vi "FipsAdjacent.vi"() -> (11 "Fips":i32[](array[numeric]))   [LabVIEW 2017] (continued)
CA\"\t06005\t\"El Dorado County, CA\"\t06017\n\"Amador County, CA\"\t06005\t\"Sacramento County, CA\"\t06067\n\"Amador County, CA\"\t06005\t\"San Joaquin County, CA\"\t06077\n\"Butte County, CA\"\t06007\t\"Butte County, CA\"\t06007\n\"Butte County, CA\"\t06007\t\"Colusa County, CA\"\t06011\n\"Butte County, CA\"\t06007\t\"Glenn County, CA\"\t06021\n\"Butte County, CA\"\t06007\t\"Plumas County, CA\"\t06063\n\"Butte County, CA\"\t06007\t\"Sutter County, CA\"\t06101\n\"Butte County, CA\"\t06007\t\"Tehama County, CA\"\t06103\n\"Butte County, CA\"\t06007\t\"Yuba County, CA\"\t06115\n\"Calaveras County, CA\"\t06009\t\"Alpine County, CA\"\t06003\n\"Calaveras County, CA\"\t06009\t\"Amador County, CA\"\t06005\n\"Calaveras County, CA\"\t06009\t\"Calaveras County, CA\"\t06009\n\"Calaveras County, CA\"\t06009\t\"San Joaquin County, CA\"\t06077\n\"Calaveras County, CA\"\t06009\t\"Stanislaus County, CA\"\t06099\n\"Calaveras County, CA\"\t06009\t\"Tuolumne County, CA\"\t06109\n\"Colusa County, CA\"\t06011\t\"Butte County, CA\"\t06007\n\"Colusa County, CA\"\t06011\t\"Colusa County, CA\"\t06011\n\"Colusa County, CA\"\t06011\t\"Glenn County, CA\"\t06021\n\"Colusa County, CA\"\t06011\t\"Lake County, CA\"\t06033\n\"Colusa County, CA\"\t06011\t\"Sutter County, CA\"\t06101\n\"Colusa County, CA\"\t06011\t\"Yolo County, CA\"\t06113\n\"Contra Costa County, CA\"\t06013\t\"Alameda County, CA\"\t06001\n\"Contra Costa County, CA\"\t06013\t\"Contra Costa County, CA\"\t06013\n\"Contra Costa County, CA\"\t06013\t\"Marin County, CA\"\t06041\n\"Contra Costa County, CA\"\t06013\t\"Sacramento County, CA\"\t06067\n\"Contra Costa County, CA\"\t06013\t\"San Francisco County, CA\"\t06075\n\"Contra Costa County, CA\"\t06013\t\"San Joaquin County, CA\"\t06077\n\"Contra Costa County, CA\"\t06013\t\"Solano County, CA\"\t06095\n\"Contra Costa County, CA\"\t06013\t\"Sonoma County, CA\"\t06097\n\"Del Norte County, CA\"\t06015\t\"Del Norte County, CA\"\t06015\n\"Del Norte County, CA\"\t06015\t\"Humboldt County, CA\"\t06023\n\"Del Norte County, CA\"\t06015\t\"Siskiyou County, CA\"\t06093\n\"Del Norte County, CA\"\t06015\t\"Curry County, OR\"\t41015\n\"Del Norte County, CA\"\t06015\t\"Josephine County, OR\"\t41033\n\"El Dorado County, CA\"\t06017\t\"Alpine County, CA\"\t06003\n\"El Dorado County, CA\"\t06017\t\"Amador County, CA\"\t06005\n\"El Dorado County, CA\"\t06017\t\"El Dorado County, CA\"\t06017\n\"El Dorado County, CA\"\t06017\t\"Placer County, CA\"\t06061\n\"El Dorado County, CA\"\t06017\t\"Sacramento County, CA\"\t06067\n\"El Dorado County, CA\"\t06017\t\"Douglas County, NV\"\t32005\n\"Fresno County, CA\"\t06019\t\"Fresno County, CA\"\t06019\n\"Fresno County, CA\"\t06019\t\"Inyo County, CA\"\t06027\n\"Fresno County, CA\"\t06019\t\"Kings County, CA\"\t06031\n\"Fresno County, CA\"\t06019\t\"Madera County, CA\"\t06039\n\"Fresno County, CA\"\t06019\t\"Merced County, CA\"\t06047\n\"Fresno County, CA\"\t06019\t\"Mono County, CA\"\t06051\n\"Fresno County, CA\"\t06019\t\"Monterey County, CA\"\t06053\n\"Fresno County, CA\"\t06019\t\"San Benito County, CA\"\t06069\n\"Fresno County, CA\"\t06019\t\"Tulare County, CA\"\t06107\n\"Glenn County, CA\"\t06021\t\"Butte County, CA\"\t06007\n\"Glenn County, CA\"\t06021\t\"Colusa County, CA\"\t06011\n\"Glenn County, CA\"\t06021\t\"Glenn County, CA\"\t06021\n\"Glenn County, CA\"\t06021\t\"Lake County, CA\"\t06033\n\"Glenn County, CA\"\t06021\t\"Mendocino County, CA\"\t06045\n\"Glenn County, CA\"\t06021\t\"Tehama County, CA\"\t06103\n\"Humboldt County, CA\"\t06023\t\"Del Norte County, CA\"\t06015\n\"Humboldt County, CA\"\t06023\t\"Humboldt County, CA\"\t06023\n\"Humboldt County, CA\"\t06023\t\"Mendocino County, CA\"\t06045\n\"Humboldt County, CA\"\t06023\t\"Siskiyou County, CA\"\t06093\n\"Humboldt County, CA\"\t06023\t\"Trinity County, CA\"\t06105\n\"Imperial County, CA\"\t06025\t\"La Paz County, AZ\"\t04012\n\"Imperial County, CA\"\t06025\t\"Yuma County, AZ\"\t04027\n\"Imperial County, CA\"\t06025\t\"Imperial County, CA\"\t06025\n\"Imperial County, CA\"\t06025\t\"Riverside County, CA\"\t06065\n\"Imperial County, CA\"\t06025\t\"San Diego County, CA\"\t06073\n\"Inyo County, CA\"\t06027\t\"Fresno County, CA\"\t06019\n\"Inyo County, CA\"\t06027\t\"Inyo County, CA\"\t06027\n\"Inyo County, CA\"\t06027\t\"Kern County, CA\"\t06029\n\"Inyo County, CA\"\t06027\t\"Mono County, CA\"\t06051\n\"Inyo County, CA\"\t06027\t\"San Bernardino County, CA\"\t06071\n\"Inyo County, CA\"\t06027\t\"Tulare County, CA\"\t06107\n\"Inyo County, CA\"\t06027\t\"Clark County, NV\"\t32003\n\"Inyo County, CA\"\t06027\t\"Esmeralda County, NV\"\t32009\n\"Inyo County, CA\"\t06027\t\"Nye County, NV\"\t32023\n\"Kern County, CA\"\t06029\t\"Inyo County, CA\"\t06027\n\"Kern County, CA\"\t06029\t\"Kern County, CA\"\t06029\n\"Kern County, CA\"\t06029\t\"Kings County, CA\"\t06031\n\"Kern County, CA\"\t06029\t\"Los Angeles County, CA\"\t06037\n\"Kern County, CA\"\t06029\t\"San Bernardino County, CA\"\t06071\n\"Kern County, CA\"\t06029\t\"San Luis Obispo County, CA\"\t06079\n\"Kern County, CA\"\t06029\t\"Santa Barbara County, CA\"\t06083\n\"Kern County, CA\"\t06029\t\"Tulare County, CA\"\t06107\n\"Kern County, CA\"\t06029\t\"Ventura County, CA\"\t06111\n\"Kings County, CA\"\t06031\t\"Fresno County, CA\"\t06019\n\"Kings County, CA\"\t06031\t\"Kern County, CA\"\t06029\n\"Kings County, CA\"\t06031\t\"Kings County, CA\"\t06031\n\"Kings County, CA\"\t06031\t\"Monterey County, CA\"\t06053\n\"Kings County, CA\"\t06031\t\"San Luis Obispo County, CA\"\t06079\n\"Kings County, CA\"\t06031\t\"Tulare County, CA\"\t06107\n\"Lake County, CA\"\t06033\t\"Colusa County, CA\"\t06011\n\"Lake County, CA\"\t06033\t\"Glenn County, CA\"\t06021\n\"Lake County, CA\"\t06033\t\"Lake County, CA\"\t06033\n\"Lake County, CA\"\t06033\t\"Mendocino County, CA\"\t06045\n\"Lake County, CA\"\t06033\t\"Napa County, CA\"\t06055\n\"Lake County, CA\"\t06033\t\"Sonoma County, CA\"\t06097\n\"Lake County, CA\"\t06033\t\"Yolo County, CA\"\t06113\n\"Lassen County, CA\"\t06035\t\"Lassen County, CA\"\t06035\n\"Lassen County, CA\"\t06035\t\"Modoc County, CA\"\t06049\n\"Lassen County, CA\"\t06035\t\"Plumas County, CA\"\t06063\n\"Lassen County, CA\"\t06035\t\"Shasta County, CA\"\t06089\n\"Lassen County, CA\"\t06035\t\"Sierra County, CA\"\t06091\n\"Lassen County, CA\"\t06035\t\"Washoe County, NV\"\t32031\n\"Los Angeles County, CA\"\t06037\t\"Kern County, CA\"\t06029\n\"Los Angeles County, CA\"\t06037\t\"Los Angeles County, CA\"\t06037\n\"Los Angeles County, CA\"\t06037\t\"Orange County, CA\"\t06059\n\"Los Angeles County, CA\"\t06037\t\"San Bernardino County, CA\"\t06071\n\"Los Angeles County, CA\"\t06037\t\"Ventura County, CA\"\t06111\n\"Madera County, CA\"\t06039\t\"Fresno County, CA\"\t06019\n\"Madera County, CA\"\t06039\t\"Madera County, CA\"\t06039\n\"Madera County, CA\"\t06039\t\"Mariposa County, CA\"\t06043\n\"Madera County, CA\"\t06039\t\"Merced County, CA\"\t06047\n\"Madera County, CA\"\t06039\t\"Mono County, CA\"\t06051\n\"Madera County, CA\"\t06039\t\"Tuolumne County, CA\"\t06109\n\"Marin County, CA\"\t06041\t\"Contra Costa County, CA\"\t06013\n\"Marin County, CA\"\t06041\t\"Marin County, CA\"\t06041\n\"Marin County, CA\"\t06041\t\"San Francisco County, CA\"\t06075\n\"Marin County, CA\"\t06041\t\"Solano County, CA\"\t06095\n\"Marin County, CA\"\t06041\t\"Sonoma County, CA\"\t06097\n\"Mariposa County, CA\"\t06043\t\"Madera County, CA\"\t06039\n\"Mariposa County, CA\"\t06043\t\"Mariposa County, CA\"\t06043\n\"Mariposa County, CA\"\t06043\t\"Merced County, CA\"\t06047\n\"Mariposa County, CA\"\t06043\t\"Stanislaus County, CA\"\t06099\n\"Mariposa County, CA\"\t06043\t\"Tuolumne County, CA\"\t06109\n\"Mendocino County, CA\"\t06045\t\"Glenn County, CA\"\t06021\n\"Mendocino County, CA\"\t06045\t\"Humboldt County, CA\"\t06023\n\"Mendocino County, CA\"\t06045\t\"Lake County, CA\"\t06033\n\"Mendocino County, CA\"\t06045\t\"Mendocino County, CA\"\t06045\n\"Mendocino County, CA\"\t06045\t\"Sonoma County, CA\"\t06097\n\"Mendocino County, CA\"\t06045\t\"Tehama County, CA\"\t06103\n\"Mendocino County, CA\"\t06045\t\"Trinity County, CA\"\t06105\n\"Merced County, CA\"\t06047\t\"Fresno County, CA\"\t06019\n\"Merced County, CA\"\t06047\t\"Madera County, CA\"\t06039\n\"Merced County, CA\"\t06047\t\"Mariposa County, CA\"\t06043\n\"Merced County, CA\"\t06047\t\"Merced County, CA\"\t06047\n\"Merced County, CA\"\t06047\t\"San Benito County, CA\"\t06069\n\"Merced County, CA\"\t06047\t\"Santa Clara County, CA\"\t06085\n\"Merced County, CA\"\t06047\t\"Stanislaus County, CA\"\t06099\n\"Modoc County, CA\"\t06049\t\"Lassen County, CA\"\t06035\n\"Modoc County, CA\"\t06049\t\"Modoc County, CA\"\t06049\n\"Modoc County, CA\"\t06049\t\"Shasta County, CA\"\t06089\n\"Modoc County, CA\"\t06049\t\"Siskiyou County, CA\"\t06093\n\"Modoc County, CA\"\t06049\t\"Washoe County, NV\"\t32031\n\"Modoc County, CA\"\t06049\t\"Klamath County, OR\"\t41035\n\"Modoc County, CA\"\t06049\t\"Lake County, OR\"\t41037\n\"Mono County, CA\"\t06051\t\"Alpine County, CA\"\t06003\n\"Mono County, CA\"\t06051\t\"Fresno County, CA\"\t06019\n\"Mono County, CA\"\t06051\t\"Inyo County, CA\"\t06027\n\"Mono County, CA\"\t06051\t\"Madera County, CA\"\t06039\n\"Mono County, CA\"\t06051\t\"Mono County, CA\"\t06051\n\"Mono County, CA\"\t06051\t\"Tuolumne County, CA\"\t06109\n\"Mono County, CA\"\t06051\t\"Douglas County, NV\"\t32005\n\"Mono County, CA\"\t06051\t\"Esmeralda County, NV\"\t32009\n\"Mono County, CA\"\t06051\t\"Lyon County, NV\"\t32019\n\"Mono County, CA\"\t06051\t\"Mineral County, NV\"\t32021\n\"Monterey County, CA\"\t06053\t\"Fresno County, CA\"\t06019\n\"Monterey County, CA\"\t06053\t\"Kings County, CA\"\t06031\n\"Monterey County, CA\"\t06053\t\"Monterey County, CA\"\t06053\n\"Monterey County, CA\"\t06053\t\"San Benito County, CA\"\t06069\n\"Monterey County, CA\"\t06053\t\"San Luis Obispo County, CA\"\t06079\n\"Monterey County, CA\"\t06053\t\"Santa Cruz County, CA\"\t06087\n\"Napa County, CA\"\t06055\t\"Lake County, CA\"\t06033\n\"Napa County, CA\"\t06055\t\"Napa County, CA\"\t06055\n\"Napa County, CA\"\t06055\t\"Solano County, CA\"\t06095\n\"Napa County, CA\"\t06055\t\"Sonoma County, CA\"\t06097\n\"Napa County, CA\"\t06055\t\"Yolo County, CA\"\t06113\n\"Nevada County, CA\"\t06057\t\"Nevada County, CA\"\t06057\n\"Nevada County, CA\"\t06057\t\"Placer County, CA\"\t06061\n\"Nevada County, CA\"\t06057\t\"Sierra County, CA\"\t06091\n\"Nevada County, CA\"\t06057\t\"Yuba County, CA\"\t06115\n\"Nevada County, CA\"\t06057\t\"Washoe County, NV\"\t32031\n\"Orange County, CA\"\t06059\t\"Los Angeles County, CA\"\t06037\n\"Orange County, CA\"\t06059\t\"Orange County, CA\"\t06059\n\"Orange County, CA\"\t06059\t\"Riverside County, CA\"\t06065\n\"Orange County, CA\"\t06059\t\"San Bernardino County, CA\"\t06071\n\"Orange County, CA\"\t06059\t\"San Diego County, CA\"\t06073\n\"Placer County, CA\"\t06061\t\"El Dorado County, CA\"\t06017\n\"Placer County, CA\"\t06061\t\"Nevada County, CA\"\t06057\n\"Placer County, CA\"\t06061\t\"Placer County, CA\"\t06061\n\"Placer County, CA\"\t06061\t\"Sacramento County, CA\"\t06067\n\"Placer County, CA\"\t06061\t\"Sutter County, CA\"\t06101\n\"Placer County, CA\"\t06061\t\"Yuba County, CA\"\t06115\n\"Placer County, CA\"\t06061\t\"Douglas County, NV\"\t32005\n\"Placer County, CA\"\t06061\t\"Washoe County, NV\"\t32031\n\"Placer County, CA\"\t06061\t\"Carson City, NV\"\t32510\n\"Plumas County, CA\"\t06063\t\"Butte County, CA\"\t06007\n\"Plumas County, CA\"\t06063\t\"Lassen County, CA\"\t06035\n\"Plumas County, CA\"\t06063\t\"Plumas County, CA\"\t06063\n\"Plumas County, CA\"\t06063\t\"Shasta County, CA\"\t06089\n\"Plumas County, CA\"\t06063\t\"Sierra County, CA\"\t06091\n\"Plumas County, CA\"\t06063\t\"Tehama County, CA\"\t06103\n\"Plumas County, CA\"\t06063\t\"Yuba County, CA\"\t06115\n\"Riverside County, CA\"\t06065\t\"La Paz County, AZ\"\t04012\n\"Riverside County, CA\"\t06065\t\"Imperial County, CA\"\t06025\n\"Riverside County, CA\"\t06065\t\"Orange County, CA\"\t06059\n\"Riverside County, CA\"\t06065\t\"Riverside County, CA\"\t06065\n\"Riverside County, CA\"\t06065\t\"San Bernardino County, CA\"\t06071\n\"Riverside County, CA\"\t06065\t\"San Diego County, CA\"\t06073\n\"Sacramento County, CA\"\t06067\t\"Amador County, CA\"\t06005\n\"Sacramento County, CA\"\t06067\t\"Contra Costa County, CA\"\t06013\n\"Sacramento County, CA\"\t06067\t\"El Dorado County, CA\"\t06017\n\"Sacramento County, CA\"\t06067\t\"Placer County, CA\"\t06061\n\"Sacramento County, CA\"\t06067\t\"Sacramento County, CA\"\t06067\n\"Sacramento County, CA\"\t06067\t\"San Joaquin County, CA\"\t06077\n\"Sacramento County, CA\"\t06067\t\"Solano County, CA\"\t06095\n\"Sacramento County, CA\"\t06067\t\"Sutter County, CA\"\t06101\n\"Sacramento County, CA\"\t06067\t\"Yolo County, CA\"\t06113\n\"San Benito County, CA\"\t06069\t\"Fresno County, CA\"\t06019\n\"San Benito County, CA\"\t06069\t\"Merced County, CA\"\t06047\n\"San Benito County, CA\"\t06069\t\"Monterey County, CA\"\t06053\n\"San Benito County, CA\"\t06069\t\"San Benito County, CA\"\t06069\n\"San Benito County, CA\"\t06069\t\"Santa Clara County, CA\"\t06085\n\"San Benito County, CA\"\t06069\t\"Santa Cruz County, CA\"\t06087\n\"San Bernardino County, CA\"\t06071\t\"La Paz County, AZ\"\t04012\n\"San Bernardino County, CA\"\t06071\t\"Mohave County, AZ\"\t04015\n\"San Bernardino County, CA\"\t06071\t\"Inyo County, CA\"\t06027\n\"San Bernardino County, CA\"\t06071\t\"Kern County, CA\"\t06029\n\"San Bernardino County, CA\"\t06071\t\"Los Angeles County, CA\"\t06037\n\"San Bernardino County, CA\"\t06071\t\"Orange County, CA\"\t06059\n\"San Bernardino County, CA\"\t06071\t\"Riverside County, CA\"\t06065\n\"San Bernardino County, CA\"\t06071\t\"San Bernardino County, CA\"\t06071\n\"San Bernardino County, CA\"\t06071\t\"Clark County, NV\"\t32003\n\"San Diego County, CA\"\t06073\t\"Imperial County, CA\"\t06025\n\"San Diego County, CA\"\t06073\t\"Orange County, CA\"\t06059\n\"San Diego County, CA\"\t06073\t\"Riverside County, CA\"\t06065\n\"San Diego County, CA\"\t06073\t\"San Diego County, CA\"\t06073\n\"San Francisco County, CA\"\t06075\t\"Alameda County, CA\"\t06001\n\"San Francisco County, CA\"\t06075\t\"Contra Costa County, CA\"\t06013\n\"San Francisco County, CA\"\t06075\t\"Marin County, CA\"\t06041\n\"San Francisco County, CA\"\t06075\t\"San Francisco County, CA\"\t06075\n\"San Francisco County, CA\"\t06075\t\"San Mateo County, CA\"\t06081\n\"San Joaquin County, CA\"\t06077\t\"Alameda County, CA\"\t06001\n\"San Joaquin County, CA\"\t06077\t\"Amador County, CA\"\t06005\n\"San Joaquin County, CA\"\t06077\t\"Calaveras County, CA\"\t06009\n\"San Joaquin County, CA\"\t06077\t\"Contra Costa County, CA\"\t06013\n\"San Joaquin County, CA\"\t06077\t\"Sacramento County, CA\"\t06067\n\"San Joaquin County, CA\"\t06077\t\"San Joaquin County, CA\"\t06077\n\"San Joaquin County, CA\"\t06077\t\"Stanislaus County, CA\"\t06099\n\"San Luis Obispo County, CA\"\t06079\t\"Kern County, CA\"\t06029\n\"San Luis Obispo County, CA\"\t06079\t\"Kings County, CA\"\t06031\n\"San Luis Obispo County, CA\"\t06079\t\"Monterey County, CA\"\t06053\n\"San Luis Obispo County, CA\"\t06079\t\"San Luis Obispo County, CA\"\t06079\n\"San Luis Obispo County, CA\"\t06079\t\"Santa Barbara County, CA\"\t06083\n\"San Mateo County, CA\"\t06081\t\"Alameda County, CA\"\t06001\n\"San Mateo County, CA\"\t06081\t\"San Francisco County, CA\"\t06075\n\"San Mateo County, CA\"\t06081\t\"San Mateo County, CA\"\t06081\n\"San Mateo County, CA\"\t06081\t\"Santa Clara County, CA\"\t06085\n\"San Mateo County, CA\"\t06081\t\"Santa Cruz County, CA\"\t06087\n\"Santa Barbara County, CA\"\t06083\t\"Kern County, CA\"\t06029\n\"Santa Barbara County, CA\"\t06083\t\"San Luis Obispo County, CA\"\t06079\n\"Santa Barbara County, CA\"\t06083\t\"Santa Barbara County, CA\"\t06083\n\"Santa Barbara County, CA\"\t06083\t\"Ventura County, CA\"\t06111\n\"Santa Clara County, CA\"\t06085\t\"Alameda County, CA\"\t06001\n\"Santa Clara County, CA\"\t06085\t\"Merced County, CA\"\t06047\n\"Santa Clara County, CA\"\t06085\t\"San Benito County, CA\"\t06069\n\"Santa Clara County, CA\"\t06085\t\"San Mateo County, CA\"\t06081\n\"Santa Clara County, CA\"\t06085\t\"Santa Clara County, CA\"\t06085\n\"Santa Clara County, CA\"\t06085\t\"Santa Cruz County, CA\"\t06087\n\"Santa Clara County, CA\"\t06085\t\"Stanislaus County, CA\"\t06099\n\"Santa Cruz County, CA\"\t06087\t\"Monterey County, CA\"\t06053\n\"Santa Cruz County, CA\"\t06087\t\"San Benito County, CA\"\t06069\n\"Santa Cruz County, CA\"\t06087\t\"San Mateo County, CA\"\t06081\n\"Santa Cruz County, CA\"\t06087\t\"Santa Clara County, CA\"\t06085\n\"Santa Cruz County, CA\"\t06087\t\"Santa Cruz County, CA\"\t06087\n\"Shasta County, CA\"\t06089\t\"Lassen County, CA\"\t06035\n\"Shasta County, CA\"\t06089\t\"Modoc County, CA\"\t06049\n\"Shasta County, CA\"\t06089\t\"Plumas County, CA\"\t06063\n\"Shasta County, CA\"\t06089\t\"Shasta County, CA\"\t06089\n\"Shasta County, CA\"\t06089\t\"Siskiyou County, CA\"\t06093\n\"Shasta County, CA\"\t06089\t\"Tehama County, CA\"\t06103\n\"Shasta County, CA\"\t06089\t\"Trinity County, CA\"\t06105\n\"Sierra County, CA\"\t06091\t\"Lassen County, CA\"\t06035\n\"Sierra County, CA\"\t06091\t\"Nevada County, CA\"\t06057\n\"Sierra County, CA\"\t06091\t\"Plumas County, CA\"\t06063\n\"Sierra County, CA\"\t06091\t\"Sierra County, CA\"\t06091\n\"Sierra County, CA\"\t06091\t\"Yuba County, CA\"\t06115\n\"Sierra County, CA\"\t06091\t\"Washoe County, NV\"\t32031\n\"Siskiyou County, CA\"\t06093\t\"Del Norte County, CA\"\t06015\n\"Siskiyou County, CA\"\t06093\t\"Humboldt County, CA\"\t06023\n\"Siskiyou County, CA\"\t06093\t\"Modoc County, CA\"\t06049\n\"Siskiyou County, CA\"\t06093\t\"Shasta County, CA\"\t06089\n\"Siskiyou County, CA\"\t06093\t\"Siskiyou County, CA\"\t06093\n\"Siskiyou County, CA\"\t06093\t\"Trinity County, CA\"\t06105\n\"Siskiyou County, CA\"\t06093\t\"Jackson County, OR\"\t41029\n\"Siskiyou County, CA\"\t06093\t\"Josephine County, OR\"\t41033\n\"Siskiyou County, CA\"\t06093\t\"Klamath County, OR\"\t41035\n\"Solano County, CA\"\t06095\t\"Contra Costa County, CA\"\t06013\n\"Solano County, CA\"\t06095\t\"Marin County, CA\"\t06041\n\"Solano County, CA\"\t06095\t\"Napa County, CA\"\t06055\n\"Solano County, CA\"\t06095\t\"Sacramento County, CA\"\t06067\n\"Solano County, CA\"\t06095\t\"Solano County, CA\"\t06095\n\"Solano County, CA\"\t06095\t\"Sonoma County, CA\"\t06097\n\"Solano County, CA\"\t06095\t\"Yolo County, CA\"\t06113\n\"Sonoma County, CA\"\t06097\t\"Contra Costa County, CA\"\t06013\n\"Sonoma County, CA\"\t06097\t\"Lake County, CA\"\t06033\n\"Sonoma County, CA\"\t06097\t\"Marin County, CA\"\t06041\n\"Sonoma County, CA\"\t06097\t\"Mendocino County, CA\"\t06045\n\"Sonoma County, CA\"\t06097\t\"Napa County, CA\"\t06055\n\"Sonoma County, CA\"\t06097\t\"Solano County, CA\"\t06095\n\"Sonoma County, CA\"\t06097\t\"Sonoma County, CA\"\t06097\n\"Stanislaus County, CA\"\t06099\t\"Alameda County, CA\"\t06001\n\"Stanislaus County, CA\"\t06099\t\"Calaveras County, CA\"\t06009\n\"Stanislaus County, CA\"\t06099\t\"Mariposa County, CA\"\t06043\n\"Stanislaus County, CA\"\t06099\t\"Merced County, CA\"\t06047\n\"Stanislaus County, CA\"\t06099\t\"San Joaquin County, CA\"\t06077\n\"Stanislaus County, CA\"\t06099\t\"Santa Clara County, CA\"\t06085\n\"Stanislaus County, CA\"\t06099\t\"Stanislaus County, CA\"\t06099\n\"Stanislaus County, CA\"\t06099\t\"Tuolumne County, CA\"\t06109\n\"Sutter County, CA\"\t06101\t\"Butte County, CA\"\t06007\n\"Sutter County, CA\"\t06101\t\"Colusa County, CA\"\t06011\n\"Sutter County, CA\"\t06101\t\"Placer County, CA\"\t06061\n\"Sutter County, CA\"\t06101\t\"Sacramento County, CA\"\t06067\n\"Sutter County, CA\"\t06101\t\"Sutter County, CA\"\t06101\n\"Sutter County, CA\"\t06101\t\"Yolo County, CA\"\t06113\n\"Sutter County, CA\"\t06101\t\"Yuba County, CA\"\t06115\n\"Tehama County, CA\"\t06103\t\"Butte County, CA\"\t06007\n\"Tehama County, CA\"\t06103\t\"Glenn County, CA\"\t06021\n\"Tehama County, CA\"\t06103\t\"Mendocino County, CA\"\t06045\n\"Tehama County, CA\"\t06103\t\"Plumas County, CA\"\t06063\n\"Tehama County, CA\"\t06103\t\"Shasta County, CA\"\t06089\n\"Tehama County, CA\"\t06103\t\"Tehama County, CA\"\t06103\n\"Tehama County, CA\"\t06103\t\"Trinity County, CA\"\t06105\n\"Trinity County, CA\"\t06105\t\"Humboldt County, CA\"\t06023\n\"Trinity County, CA\"\t06105\t\"Mendocino County, CA\"\t06045\n\"Trinity County, CA\"\t06105\t\"Shasta County, CA\"\t06089\n\"Trinity County, CA\"\t06105\t\"Siskiyou County, CA\"\t06093\n\"Trinity County, CA\"\t06105\t\"Tehama County, CA\"\t06103\n\"Trinity County, CA\"\t06105\t\"Trinity County, CA\"\t06105\n\"Tulare County, CA\"\t06107\t\"Fresno County, CA\"\t06019\n\"Tulare County, CA\"\t06107\t\"Inyo County, CA\"\t06027\n\"Tulare County, CA\"\t06107\t\"Kern County, CA\"\t06029\n\"Tulare County, CA\"\t06107\t\"Kings County, CA\"\t06031\n\"Tulare County, CA\"\t06107\t\"Tulare County, CA\"\t06107\n\"Tuolumne County, CA\"\t06109\t\"Alpine County, CA\"\t06003\n\"Tuolumne County, CA\"\t06109\t\"Calaveras County, CA\"\t06009\n\"Tuolumne County, CA\"\t06109\t\"Madera County, CA\"\t06039\n\"Tuolumne County, CA\"\t06109\t\"Mariposa County, CA\"\t06043\n\"Tuolumne County, CA\"\t06109\t\"Mono County, CA\"\t06051\n\"Tuolumne County, CA\"\t06109\t\"Stanislaus County, CA\"\t06099\n\"Tuolumne County, CA\"\t06109\t\"Tuolumne County, CA\"\t06109\n\"Ventura County, CA\"\t06111\t\"Kern County, CA\"\t06029\n\"Ventura County, CA\"\t06111\t\"Los Angeles County, CA\"\t06037\n\"Ventura County, CA\"\t06111\t\"Santa Barbara County, CA\"\t06083\n\"Ventura County, CA\"\t06111\t\"Ventura County, CA\"\t06111\n\"Yolo County, CA\"\t06113\t\"Colusa County, CA\"\t06011\n\"Yolo County, CA\"\t06113\t\"Lake County, CA\"\t06033\n\"Yolo County, CA\"\t06113\t\"Napa County, CA\"\t06055\n\"Yolo County, CA\"\t06113\t\"Sacramento County, CA\"\t06067\n\"Yolo County, CA\"\t06113\t\"Solano County, CA\"\t06095\n\"Yolo County, CA\"\t06113\t\"Sutter County, CA\"\t06101\n\"Yolo County, CA\"\t06113\t\"Yolo County, CA\"\t06113\n\"Yuba County, CA\"\t06115\t\"Butte County, CA\"\t06007\n\"Yuba County, CA\"\t06115\t\"Nevada County, CA\"\t06057\n\"Yuba County, CA\"\t06115\t\"Placer County, CA\"\t06061\n\"Yuba County, CA\"\t06115\t\"Plumas County, CA\"\t06063\n\"Yuba County, CA\"\t06115\t\"Sierra County, CA\"\t06091\n\"Yuba County, CA\"\t06115\t\"Sutter County, CA\"\t06101\n\"Yuba County, CA\"\t06115\t\"Yuba County, CA\"\t06115\n\"Adams County, CO\"\t08001\t\"Adams County, CO\"\t08001\n\"Adams County, CO\"\t08001\t\"Arapahoe County, CO\"\t08005\n\"Adams County, CO\"\t08001\t\"Broomfield County, CO\"\t08014\n\"Adams County, CO\"\t08001\t\"Denver County, CO\"\t08031\n\"Adams County, CO\"\t08001\t\"Jefferson County, CO\"\t08059\n\"Adams County, CO\"\t08001\t\"Morgan County, CO\"\t08087\n\"Adams County, CO\"\t08001\t\"Washington County, CO\"\t08121\n\"Adams County, CO\"\t08001\t\"Weld County, CO\"\t08123\n\"Alamosa County, CO\"\t08003\t\"Alamosa County, CO\"\t08003\n\"Alamosa County, CO\"\t08003\t\"Conejos County, CO\"\t08021\n\"Alamosa County, CO\"\t08003\t\"Costilla County, CO\"\t08023\n\"Alamosa County, CO\"\t08003\t\"Huerfano County, CO\"\t08055\n\"Alamosa County, CO\"\t08003\t\"Rio Grande County, CO\"\t08105\n\"Alamosa County, CO\"\t08003\t\"Saguache County, CO\"\t08109\n\"Arapahoe County, CO\"\t08005\t\"Adams County, CO\"\t08001\n\"Arapahoe County, CO\"\t08005\t\"Arapahoe County, CO\"\t08005\n\"Arapahoe County, CO\"\t08005\t\"Denver County, CO\"\t08031\n\"Arapahoe County, CO\"\t08005\t\"Douglas County, CO\"\t08035\n\"Arapahoe County, CO\"\t08005\t\"Elbert County, CO\"\t08039\n\"Arapahoe County, CO\"\t08005\t\"Jefferson County, CO\"\t08059\n\"Arapahoe County, CO\"\t08005\t\"Lincoln County, CO\"\t08073\n\"Arapahoe County, CO\"\t08005\t\"Washington County, CO\"\t08121\n\"Archuleta County, CO\"\t08007\t\"Archuleta County, CO\"\t08007\n\"Archuleta County, CO\"\t08007\t\"Conejos County, CO\"\t08021\n\"Archuleta County, CO\"\t08007\t\"Hinsdale County, CO\"\t08053\n\"Archuleta County, CO\"\t08007\t\"La Plata County, CO\"\t08067\n\"Archuleta County, CO\"\t08007\t\"Mineral County, CO\"\t08079\n\"Archuleta County, CO\"\t08007\t\"Rio Grande County, CO\"\t08105\n\"Archuleta County, CO\"\t08007\t\"Rio Arriba County, NM\"\t35039\n\"Archuleta County, CO\"\t08007\t\"San Juan County, NM\"\t35045\n\"Baca County, CO\"\t08009\t\"Baca County, CO\"\t08009\n\"Baca County, CO\"\t08009\t\"Bent County, CO\"\t08011\n\"Baca County, CO\"\t08009\t\"Las Animas County, CO\"\t08071\n\"Baca County, CO\"\t08009\t\"Prowers County, CO\"\t08099\n\"Baca County, CO\"\t08009\t\"Morton County, KS\"\t20129\n\"Baca County, CO\"\t08009\t\"Stanton County, KS\"\t20187\n\"Baca County, CO\"\t08009\t\"Union County, NM\"\t35059\n\"Baca County, CO\"\t08009\t\"Cimarron County, OK\"\t40025\n\"Bent County, CO\"\t08011\t\"Baca County, CO\"\t08009\n\"Bent County, CO\"\t08011\t\"Bent County, CO\"\t08011\n\"Bent County, CO\"\t08011\t\"Kiowa County, CO\"\t08061\n\"Bent County, CO\"\t08011\t\"Las Animas County, CO\"\t08071\n\"Bent County, CO\"\t08011\t\"Otero County, CO\"\t08089\n\"Bent County, CO\"\t08011\t\"Prowers County, CO\"\t08099\n\"Boulder County, CO\"\t08013\t\"Boulder County, CO\"\t08013\n\"Boulder County, CO\"\t08013\t\"Broomfield County, CO\"\t08014\n\"Boulder County, CO\"\t08013\t\"Gilpin County, CO\"\t08047\n\"Boulder County, CO\"\t08013\t\"Grand County, CO\"\t08049\n\"Boulder County, CO\"\t08013\t\"Jefferson County, CO\"\t08059\n\"Boulder County, CO\"\t08013\t\"Larimer County, CO\"\t08069\n\"Boulder County, CO\"\t08013\t\"Weld County, CO\"\t08123\n\"Broomfield County, CO\"\t08014\t\"Adams County, CO\"\t08001\n\"Broomfield County, CO\"\t08014\t\"Boulder County, CO\"\t08013\n\"Broomfield County, CO\"\t08014\t\"Broomfield County, CO\"\t08014\n\"Broomfield County, CO\"\t08014\t\"Jefferson County, CO\"\t08059\n\"Broomfield County, CO\"\t08014\t\"Weld County, CO\"\t08123\n\"Chaffee County, CO\"\t08015\t\"Chaffee County, CO\"\t08015\n\"Chaffee County, CO\"\t08015\t\"Fremont County, CO\"\t08043\n\"Chaffee County, CO\"\t08015\t\"Gunnison County, CO\"\t08051\n\"Chaffee County, CO\"\t08015\t\"Lake County, CO\"\t08065\n\"Chaffee County, CO\"\t08015\t\"Park County, CO\"\t08093\n\"Chaffee County, CO\"\t08015\t\"Pitkin County, CO\"\t08097\n\"Chaffee County, CO\"\t08015\t\"Saguache County, CO\"\t08109\n\"Cheyenne County, CO\"\t08017\t\"Cheyenne County, CO\"\t08017\n\"Cheyenne County, CO\"\t08017\t\"Kiowa County, CO\"\t08061\n\"Cheyenne County, CO\"\t08017\t\"Kit Carson County, CO\"\t08063\n\"Cheyenne County, CO\"\t08017\t\"Lincoln County, CO\"\t08073\n\"Cheyenne County, CO\"\t08017\t\"Greeley County, KS\"\t20071\n\"Cheyenne County, CO\"\t08017\t\"Wallace County, KS\"\t20199\n\"Clear Creek County, CO\"\t08019\t\"Clear Creek County, CO\"\t08019\n\"Clear Creek County, CO\"\t08019\t\"Gilpin County, CO\"\t08047\n\"Clear Creek County, CO\"\t08019\t\"Grand County, CO\"\t08049\n\"Clear Creek County, CO\"\t08019\t\"Jefferson County, CO\"\t08059\n\"Clear Creek County, CO\"\t08019\t\"Park County, CO\"\t08093\n\"Clear Creek County, CO\"\t08019\t\"Summit County, CO\"\t08117\n\"Conejos County, CO\"\t08021\t\"Alamosa County, CO\"\t08003\n\"Conejos County, CO\"\t08021\t\"Archuleta County, CO\"\t08007\n\"Conejos County, CO\"\t08021\t\"Conejos County, CO\"\t08021\n\"Conejos County, CO\"\t08021\t\"Costilla County, CO\"\t08023\n\"Conejos County, CO\"\t08021\t\"Rio Grande County, CO\"\t08105\n\"Conejos County, CO\"\t08021\t\"Rio Arriba County, NM\"\t35039\n\"Conejos County, CO\"\t08021\t\"Taos County, NM\"\t35055\n\"Costilla County, CO\"\t08023\t\"Alamosa County, CO\"\t08003\n\"Costilla County, CO\"\t08023\t\"Conejos County, CO\"\t08021\n\"Costilla County, CO\"\t08023\t\"Costilla County, CO\"\t08023\n\"Costilla County, CO\"\t08023\t\"Huerfano County, CO\"\t08055\n\"Costilla County, CO\"\t08023\t\"Las Animas County, CO\"\t08071\n\"Costilla County, CO\"\t08023\t\"Colfax County, NM\"\t35007\n\"Costilla County, CO\"\t08023\t\"Taos County, NM\"\t35055\n\"Crowley County, CO\"\t08025\t\"Crowley County, CO\"\t08025\n\"Crowley County, CO\"\t08025\t\"El Paso County, CO\"\t08041\n\"Crowley County, CO\"\t08025\t\"Kiowa County, CO\"\t08061\n\"Crowley County, CO\"\t08025\t\"Lincoln County, CO\"\t08073\n\"Crowley County, CO\"\t08025\t\"Otero County, CO\"\t08089\n\"Crowley County, CO\"\t08025\t\"Pueblo County, CO\"\t08101\n\"Custer County, CO\"\t08027\t\"Custer County, CO\"\t08027\n\"Custer County, CO\"\t08027\t\"Fremont County, CO\"\t08043\n\"Custer County, CO\"\t08027\t\"Huerfano County, CO\"\t08055\n\"Custer County, CO\"\t08027\t\"Pueblo County, CO\"\t08101\n\"Custer County, CO\"\t08027\t\"Saguache County, CO\"\t08109\n\"Delta County, CO\"\t08029\t\"Delta County, CO\"\t08029\n\"Delta County, CO\"\t08029\t\"Gunnison County, CO\"\t08051\n\"Delta County, CO\"\t08029\t\"Mesa County, CO\"\t08077\n\"Delta County, CO\"\t08029\t\"Montrose County, CO\"\t08085\n\"Denver County, CO\"\t08031\t\"Adams County, CO\"\t08001\n\"Denver County, CO\"\t08031\t\"Arapahoe County, CO\"\t08005\n\"Denver County, CO\"\t08031\t\"Denver County, CO\"\t08031\n\"Denver County, CO\"\t08031\t\"Jefferson County, CO\"\t08059\n\"Dolores County, CO\"\t08033\t\"Dolores County, CO\"\t08033\n\"Dolores County, CO\"\t08033\t\"La Plata County, CO\"\t08067\n\"Dolores County, CO\"\t08033\t\"Montezuma County, CO\"\t08083\n\"Dolores County, CO\"\t08033\t\"San Juan County, CO\"\t08111\n\"Dolores County, CO\"\t08033\t\"San Miguel County, CO\"\t08113\n\"Dolores County, CO\"\t08033\t\"San Juan County, UT\"\t49037\n\"Douglas County, CO\"\t08035\t\"Arapahoe County, CO\"\t08005\n\"Douglas County, CO\"\t08035\t\"Douglas County, CO\"\t08035\n\"Douglas County, CO\"\t08035\t\"Elbert County, CO\"\t08039\n\"Douglas County, CO\"\t08035\t\"El Paso County, CO\"\t08041\n\"Douglas County, CO\"\t08035\t\"Jefferson County, CO\"\t08059\n\"Douglas County, CO\"\t08035\t\"Teller County, CO\"\t08119\n\"Eagle County, CO\"\t08037\t\"Eagle County, CO\"\t08037\n\"Eagle County, CO\"\t08037\t\"Garfield County, CO\"\t08045\n\"Eagle County, CO\"\t08037\t\"Grand County, CO\"\t08049\n\"Eagle County, CO\"\t08037\t\"Lake County, CO\"\t08065\n\"Eagle County, CO\"\t08037\t\"Pitkin County, CO\"\t08097\n\"Eagle County, CO\"\t08037\t\"Routt County, CO\"\t08107\n\"Eagle County, CO\"\t08037\t\"Summit County, CO\"\t08117\n\"Elbert County, CO\"\t08039\t\"Arapahoe County, CO\"\t08005\n\"Elbert County, CO\"\t08039\t\"Douglas County, CO\"\t08035\n\"Elbert County, CO\"\t08039\t\"Elbert County, CO\"\t08039\n\"Elbert County, CO\"\t08039\t\"El Paso County, CO\"\t08041\n\"Elbert County, CO\"\t08039\t\"Lincoln County, CO\"\t08073\n\"El Paso County, CO\"\t08041\t\"Crowley County, CO\"\t08025\n\"El Paso County, CO\"\t08041\t\"Douglas County, CO\"\t08035\n\"El Paso County, CO\"\t08041\t\"Elbert County, CO\"\t08039\n\"El Paso County, CO\"\t08041\t\"El Paso County, CO\"\t08041\n\"El Paso County, CO\"\t08041\t\"Fremont County, CO\"\t08043\n\"El Paso County, CO\"\t08041\t\"Lincoln County, CO\"\t08073\n\"El Paso County, CO\"\t08041\t\"Pueblo County, CO\"\t08101\n\"El Paso County, CO\"\t08041\t\"Teller County, CO\"\t08119\n\"Fremont County, CO\"\t08043\t\"Chaffee County, CO\"\t08015\n\"Fremont County, CO\"\t08043\t\"Custer County, CO\"\t08027\n\"Fremont County, CO\"\t08043\t\"El Paso County, CO\"\t08041\n\"Fremont County, CO\"\t08043\t\"Fremont County, CO\"\t08043\n\"Fremont County, CO\"\t08043\t\"Park County, CO\"\t08093\n\"Fremont County, CO\"\t08043\t\"Pueblo County, CO\"\t08101\n\"Fremont County, CO\"\t08043\t\"Saguache County, CO\"\t08109\n\"Fremont County, CO\"\t08043\t\"Teller County, CO\"\t08119\n\"Garfield County, CO\"\t08045\t\"Eagle County, CO\"\t08037\n\"Garfield County, CO\"\t08045\t\"Garfield County, CO\"\t08045\n\"Garfield County, CO\"\t08045\t\"Mesa County, CO\"\t08077\n\"Garfield County, CO\"\t08045\t\"Pitkin County, CO\"\t08097\n\"Garfield County, CO\"\t08045\t\"Rio Blanco County, CO\"\t08103\n\"Garfield County, CO\"\t08045\t\"Routt County, CO\"\t08107\n\"Garfield County, CO\"\t08045\t\"Grand County, UT\"\t49019\n\"Garfield County, CO\"\t08045\t\"Uintah County, UT\"\t49047\n\"Gilpin County, CO\"\t08047\t\"Boulder County, CO\"\t08013\n\"Gilpin County, CO\"\t08047\t\"Clear Creek County, CO\"\t08019\n\"Gilpin County, CO\"\t08047\t\"Gilpin County, CO\"\t08047\n\"Gilpin County, CO\"\t08047\t\"Grand County, CO\"\t08049\n\"Gilpin County, CO\"\t08047\t\"Jefferson County, CO\"\t08059\n\"Grand County, CO\"\t08049\t\"Boulder County, CO\"\t08013\n\"Grand County, CO\"\t08049\t\"Clear Creek County, CO\"\t08019\n\"Grand County, CO\"\t08049\t\"Eagle County, CO\"\t08037\n\"Grand County, CO\"\t08049\t\"Gilpin County, CO\"\t08047\n\"Grand County, CO\"\t08049\t\"Grand County, CO\"\t08049\n\"Grand County, CO\"\t08049\t\"Jackson County, CO\"\t08057\n\"Grand County, CO\"\t08049\t\"Larimer County, CO\"\t08069\n\"Grand County, CO\"\t08049\t\"Routt County, CO\"\t08107\n\"Grand County, CO\"\t08049\t\"Summit County, CO\"\t08117\n\"Gunnison County, CO\"\t08051\t\"Chaffee County, CO\"\t08015\n\"Gunnison County, CO\"\t08051\t\"Delta County, CO\"\t08029\n\"Gunnison County, CO\"\t08051\t\"Gunnison County, CO\"\t08051\n\"Gunnison County, CO\"\t08051\t\"Hinsdale County, CO\"\t08053\n\"Gunnison County, CO\"\t08051\t\"Mesa County, CO\"\t08077\n\"Gunnison County, CO\"\t08051\t\"Montrose County, CO\"\t08085\n\"Gunnison County, CO\"\t08051\t\"Ouray County, CO\"\t08091\n\"Gunnison County, CO\"\t08051\t\"Pitkin County, CO\"\t08097\n\"Gunnison County, CO\"\t08051\t\"Saguache County, CO\"\t08109\n\"Hinsdale County, CO\"\t08053\t\"Archuleta County, CO\"\t08007\n\"Hinsdale County, CO\"\t08053\t\"Gunnison County, CO\"\t08051\n\"Hinsdale County, CO\"\t08053\t\"Hinsdale County, CO\"\t08053\n\"Hinsdale County, CO\"\t08053\t\"La Plata County, CO\"\t08067\n\"Hinsdale County, CO\"\t08053\t\"Mineral County, CO\"\t08079\n\"Hinsdale County, CO\"\t08053\t\"Ouray County, CO\"\t08091\n\"Hinsdale County, CO\"\t08053\t\"Saguache County, CO\"\t08109\n\"Hinsdale County, CO\"\t08053\t\"San Juan County, CO\"\t08111\n\"Huerfano County, CO\"\t08055\t\"Alamosa County, CO\"\t08003\n\"Huerfano County, CO\"\t08055\t\"Costilla County, CO\"\t08023\n\"Huerfano County, CO\"\t08055\t\"Custer County, CO\"\t08027\n\"Huerfano County, CO\"\t08055\t\"Huerfano County, CO\"\t08055\n\"Huerfano County, CO\"\t08055\t\"Las Animas County, CO\"\t08071\n\"Huerfano County, CO\"\t08055\t\"Pueblo County, CO\"\t08101\n\"Huerfano County, CO\"\t08055\t\"Saguache County, CO\"\t08109\n\"Jackson County, CO\"\t08057\t\"Grand County, CO\"\t08049\n\"Jackson County, CO\"\t08057\t\"Jackson County, CO\"\t08057\n\"Jackson County, CO\"\t08057\t\"Larimer County, CO\"\t08069\n\"Jackson County, CO\"\t08057\t\"Routt County, CO\"\t08107\n\"Jackson County, CO\"\t08057\t\"Albany County, WY\"\t56001\n\"Jackson County, CO\"\t08057\t\"Carbon County, WY\"\t56007\n\"Jefferson County, CO\"\t08059\t\"Adams County, CO\"\t08001\n\"Jefferson County, CO\"\t08059\t\"Arapahoe County, CO\"\t08005\n\"Jefferson County, CO\"\t08059\t\"Boulder County, CO\"\t08013\n\"Jefferson County, CO\"\t08059\t\"Broomfield County, CO\"\t08014\n\"Jefferson County, CO\"\t08059\t\"Clear Creek County, CO\"\t08019\n\"Jefferson County, CO\"\t08059\t\"Denver County, CO\"\t08031\n\"Jefferson County, CO\"\t08059\t\"Douglas County, CO\"\t08035\n\"Jefferson County, CO\"\t08059\t\"Gilpin County, CO\"\t08047\n\"Jefferson County, CO\"\t08059\t\"Jefferson County, CO\"\t08059\n\"Jefferson County, CO\"\t08059\t\"Park County, CO\"\t08093\n\"Jefferson County, CO\"\t08059\t\"Teller County, CO\"\t08119\n\"Kiowa County, CO\"\t08061\t\"Bent County, CO\"\t08011\n\"Kiowa County, CO\"\t08061\t\"Cheyenne County, CO\"\t08017\n\"Kiowa County, CO\"\t08061\t\"Crowley County, CO\"\t08025\n\"Kiowa County, CO\"\t08061\t\"Kiowa County, CO\"\t08061\n\"Kiowa County, CO\"\t08061\t\"Lincoln County, CO\"\t08073\n\"Kiowa County, CO\"\t08061\t\"Otero County, CO\"\t08089\n\"Kiowa County, CO\"\t08061\t\"Prowers County, CO\"\t08099\n\"Kiowa County, CO\"\t08061\t\"Greeley County, KS\"\t20071\n\"Kit Carson County, CO\"\t08063\t\"Cheyenne County, CO\"\t08017\n\"Kit Carson County, CO\"\t08063\t\"Kit Carson County, CO\"\t08063\n\"Kit Carson County, CO\"\t08063\t\"Lincoln County, CO\"\t08073\n\"Kit Carson County, CO\"\t08063\t\"Washington County, CO\"\t08121\n\"Kit Carson County, CO\"\t08063\t\"Yuma County, CO\"\t08125\n\"Kit Carson County, CO\"\t08063\t\"Cheyenne County, KS\"\t20023\n\"Kit Carson County, CO\"\t08063\t\"Sherman County, KS\"\t20181\n\"Kit Carson County, CO\"\t08063\t\"Wallace County, KS\"\t20199\n\"Lake County, CO\"\t08065\t\"Chaffee County, CO\"\t08015\n\"Lake County, CO\"\t08065\t\"Eagle County, CO\"\t08037\n\"Lake County, CO\"\t08065\t\"Lake County, CO\"\t08065\n\"Lake County, CO\"\t08065\t\"Park County, CO\"\t08093\n\"Lake County, CO\"\t08065\t\"Pitkin County, CO\"\t08097\n\"Lake County, CO\"\t08065\t\"Summit County, CO\"\t08117\n\"La Plata County, CO\"\t08067\t\"Archuleta County, CO\"\t08007\n\"La Plata County, CO\"\t08067\t\"Dolores County, CO\"\t08033\n\"La Plata County, CO\"\t08067\t\"Hinsdale County, CO\"\t08053\n\"La Plata County, CO\"\t08067\t\"La Plata County, CO\"\t08067\n\"La Plata County, CO\"\t08067\t\"Montezuma County, CO\"\t08083\n\"La Plata County, CO\"\t08067\t\"San Juan County, CO\"\t08111\n\"La Plata County, CO\"\t08067\t\"San Juan County, NM\"\t35045\n\"Larimer County, CO\"\t08069\t\"Boulder County, CO\"\t08013\n\"Larimer County, CO\"\t08069\t\"Grand County, CO\"\t08049\n\"Larimer County, CO\"\t08069\t\"Jackson County, CO\"\t08057\n\"Larimer County, CO\"\t08069\t\"Larimer County, CO\"\t08069\n\"Larimer County, CO\"\t08069\t\"Weld County, CO\"\t08123\n\"Larimer County, CO\"\t08069\t\"Albany County, WY\"\t56001\n\"Larimer County, CO\"\t08069\t\"Laramie County, WY\"\t56021\n\"Las Animas County, CO\"\t08071\t\"Baca County, CO\"\t08009\n\"Las Animas County, CO\"\t08071\t\"Bent County, CO\"\t08011\n\"Las Animas County, CO\"\t08071\t\"Costilla County, CO\"\t08023\n\"Las Animas County, CO\"\t08071\t\"Huerfano County, CO\"\t08055\n\"Las Animas County, CO\"\t08071\t\"Las Animas County, CO\"\t08071\n\"Las Animas County, CO\"\t08071\t\"Otero County, CO\"\t08089\n\"Las Animas County, CO\"\t08071\t\"Pueblo County, CO\"\t08101\n\"Las Animas County, CO\"\t08071\t\"Colfax County, NM\"\t35007\n\"Las Animas County, CO\"\t08071\t\"Union County, NM\"\t35059\n\"Lincoln County, CO\"\t08073\t\"Arapahoe County, CO\"\t08005\n\"Lincoln County, CO\"\t08073\t\"Cheyenne County, CO\"\t08017\n\"Lincoln County, CO\"\t08073\t\"Crowley County, CO\"\t08025\n\"Lincoln County, CO\"\t08073\t\"Elbert County, CO\"\t08039\n\"Lincoln County, CO\"\t08073\t\"El Paso County, CO\"\t08041\n\"Lincoln County, CO\"\t08073\t\"Kiowa County, CO\"\t08061\n\"Lincoln County, CO\"\t08073\t\"Kit Carson County, CO\"\t08063\n\"Lincoln County, CO\"\t08073\t\"Lincoln County, CO\"\t08073\n\"Lincoln County, CO\"\t08073\t\"Pueblo County, CO\"\t08101\n\"Lincoln County, CO\"\t08073\t\"Washington County, CO\"\t08121\n\"Logan County, CO\"\t08075\t\"Logan County, CO\"\t08075\n\"Logan County, CO\"\t08075\t\"Morgan County, CO\"\t08087\n\"Logan County, CO\"\t08075\t\"Phillips County, CO\"\t08095\n\"Logan County, CO\"\t08075\t\"Sedgwick County, CO\"\t08115\n\"Logan County, CO\"\t08075\t\"Washington County, CO\"\t08121\n\"Logan County, CO\"\t08075\t\"Weld County, CO\"\t08123\n\"Logan County, CO\"\t08075\t\"Yuma County, CO\"\t08125\n\"Logan County, CO\"\t08075\t\"Cheyenne County, NE\"\t31033\n\"Logan County, CO\"\t08075\t\"Kimball County, NE\"\t31105\n\"Mesa County, CO\"\t08077\t\"Delta County, CO\"\t08029\n\"Mesa County, CO\"\t08077\t\"Garfield County, CO\"\t08045\n\"Mesa County, CO\"\t08077\t\"Gunnison County, CO\"\t08051\n\"Mesa County, CO\"\t08077\t\"Mesa County, CO\"\t08077\n\"Mesa County, CO\"\t08077\t\"Montrose County, CO\"\t08085\n\"Mesa County, CO\"\t08077\t\"Pitkin County, CO\"\t08097\n\"Mesa County, CO\"\t08077\t\"Grand County, UT\"\t49019\n\"Mesa County, CO\"\t08077\t\"San Juan County, UT\"\t49037\n\"Mineral County, CO\"\t08079\t\"Archuleta County, CO\"\t08007\n\"Mineral County, CO\"\t
